vi "HP81110A Set Trigger Count.vi"(8 "error in (no error)":errorcluster, 10 "Trigger Count":i32, 11 "VISA session":refnum<visa-resource-name>) -> (0 "error out":errorcluster, 3 "dup VISA session":refnum<visa-resource-name>)   [LabVIEW 2009]
doc: "This VI queries the \"trigger counts\" which correspond to the number of pulses per \"trigger\" (aka arm).\nThe number of trigger counts is returned. Also, the mode is returned, intrepreted as follows:\n0 = Pulsed (1 trigger count)\n1 = Pattern (more than 1 trigger count)"
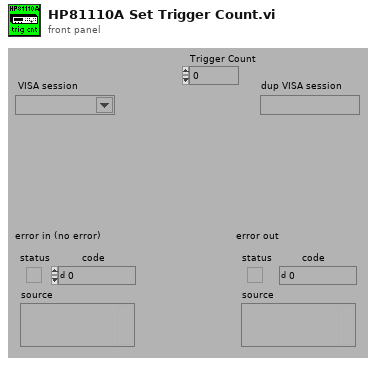
[diagram p1: front panel]
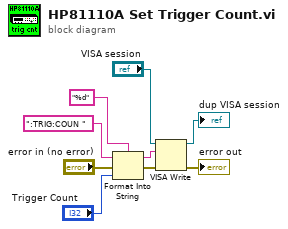
[diagram p0: block diagram]
diagram:
  n1 = Format Into String(format string="%d", initial string=":TRIG:COUN ", error in="error in (no error)", "Trigger Count") -> (resulting string=w5:string, error out=w3:errorcluster)
  n2 = VISA Write(VISA resource name="VISA session", write buffer=w5, error in (no error)=w3) -> (VISA resource name out=→"dup VISA session":refnum<visa-resource-name>, error out=→"error out":errorcluster)  [unwired: 1 out]
